vi "Who's Driver.vi"(11 "input cluster":T1) -> (2 "Yout":dbl, 3 "Xout":dbl)   [LabVIEW 2016]
uses:
  Controls.ctl
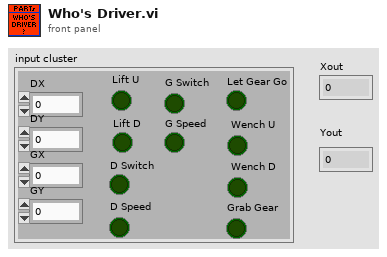
[diagram p1: front panel]
types:
  T1 = typedef "Controls.ctl" = cluster{"DX":dbl, "DY":dbl, "GX":dbl, "GY":dbl, "Lift U":bool, "D Switch":bool, "D Speed":bool, "G Switch":bool, "G Speed":bool, " Wench U":bool, " Wench D":bool, "Lift D":bool, "Let Gear Go":bool, "Grab Gear":bool}
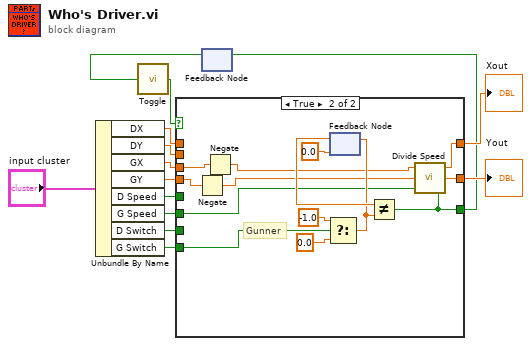
[diagram p0: block diagram]
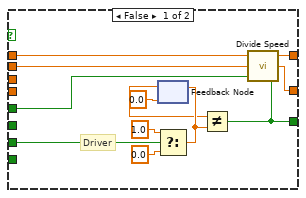
[diagram p2: hidden frame]
diagram:
  n1 = Unbundle By Name("input cluster") -> ("DX"=w3:dbl, "DY"=w4:dbl, "GX"=w5:dbl, "GY"=w6:dbl, "D Speed"=w11:bool, "G Speed"=w12:bool, "D Switch"=w2:bool, "G Switch"=w1:bool)
  n2 = feedback #1() -> (w9:bool)  [unwired: 1 in]
  n3 = call "Toggle.vi"("Input"=w9) -> ("Output"=w8:bool)  [unwired: 4 in]
  n4 = case shown="True" w8 {
    tunnel: [w16 w32] -> w7
    tunnel: w3 -> [w21 _]
    tunnel: w4 -> [w20 _]
    tunnel: w5 -> [_ w27]
    tunnel: w6 -> [_ w29]
    tunnel: [w19 w35] -> w13
    tunnel: [w18 w34] -> w14
    tunnel: w11 -> [w17 _]
    tunnel: w12 -> [_ w33]
    tunnel: w2 -> [w15 _]
    tunnel: w1 -> [_ w31]
    frame False {
      # "Driver"
      n5 = feedback #2(0.0 ("t")) -> (w25:dbl)
      n6 = Select(t=1.0, s=w15, f=0.0) -> (s? t:f=w26:dbl)
      n7 = feedback-in #2(w26) -> ()
      n8 = Not Equal?(x=w25, y=w26) -> (x != y?=w16:bool)
      n9 = call "Divide Speed.vi"("Reset"=w16, "Speed"=w17, "Y"=w20, "X"=w21) -> ("Yout"=w18:dbl, "Xout"=w19:dbl)
    }
    frame True {
      # "Gunner"
      n10 = Negate(x=w29) -> (-x=w28:dbl)
      n11 = Negate(x=w27) -> (-x=w30:dbl)
      n12 = Select(t=-1.0, s=w31, f=0.0) -> (s? t:f=w36:dbl)
      n13 = feedback #3(0.0 ("t")) -> (w37:dbl)
      n14 = feedback-in #3(w36) -> ()
      n15 = Not Equal?(x=w37, y=w36) -> (x != y?=w32:bool)
      n16 = call "Divide Speed.vi"("Reset"=w32, "Speed"=w33, "Y"=w28, "X"=w30) -> ("Yout"=w34:dbl, "Xout"=w35:dbl)
    }
  }
  "Yout" <- w14
  "Xout" <- w13
  n17 = feedback-in #1(w7) -> ()
